vi "PWM Start.vi"(9 "RunTimeUs":u32, 10 "ChannelMask":u8, 11 "DevHandle":i32) -> (3 "function return":i32)   [LabVIEW 2010, in "usb2pwm.lvlib"]
doc: "int WINAPI PWM_Start(int DevHandle,unsigned char ChannelMask,unsigned int RunTimeUs);"
uses:
  usb2pwm.lvlib
  USB2XXX.dll
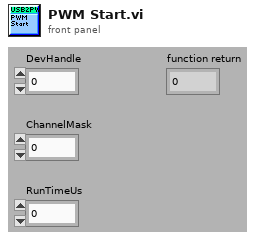
[diagram p1: front panel]
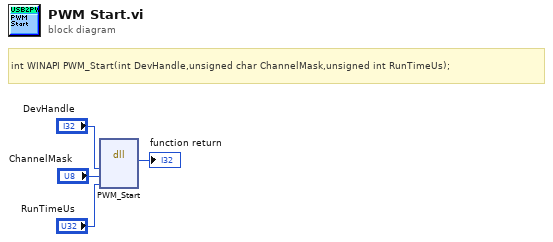
[diagram p0: block diagram]
diagram:
  # "int WINAPI PWM_Start(int DevHandle,unsigned char ChannelMask,unsigned int RunTimeUs);"
  n1 = dll-call lib="G:/OtherWork/USB2XXX_Example/trunk/Labview/PublicFiles/USB2XXX.*" fn="PWM_Start"("DevHandle"="DevHandle", "ChannelMask"="ChannelMask", "RunTimeUs"="RunTimeUs") -> (→"function return":i32)  [unwired: 6 in, 2 out]
